vi "rd_data (WFM).vi"(4 "record index":u32, 6 "record info":T3, 7 "recordLenFromStart":u64, 8 "error in (no error)":errorcluster, 9 "length":u64, 10 "record start":u64, 11 "ExcelRefnum":T4) -> (0 "error out":errorcluster, 2 "data_AllTypeData":T1, 3 "real length":u64)   [LabVIEW 2020, in "NI_ExcelFile.lvlib"]
uses:
  <vilib>/express/express shared/NI_ExcelFile/NI_ExcelFile.lvlib
  <vilib>/express/express shared/NI_ExcelFile/Ctrls/ExcelRefnum.ctl
  <vilib>/express/express shared/NI_ExcelFile/Ctrls/MainData.ctl
  <vilib>/express/express shared/NI_ExcelFile/Ctrls/StreamMode.ctl
  <vilib>/express/express shared/NI_ExcelFile/Ctrls/TimeColumnMode.ctl
  <vilib>/express/express shared/NI_ExcelFile/Ctrls/FileAttribute.ctl
  <vilib>/express/express shared/NI_ExcelFile/Ctrls/Columns.ctl
  <vilib>/express/express shared/NI_ExcelFile/Ctrls/ColumnInfo.ctl
  <vilib>/express/express shared/NI_ExcelFile/Ctrls/DataType.ctl
  <vilib>/express/express shared/NI_ExcelFile/Ctrls/wd_recordInfo.ctl
  <vilib>/express/express shared/NI_ExcelFile/Ctrls/disk_TemplateFile.ctl
  <vilib>/express/express shared/NI_ExcelFile/Ctrls/meta_file.ctl
  <vilib>/express/express shared/NI_ExcelFile/Ctrls/meta_Block.ctl
  <vilib>/express/express shared/NI_ExcelFile/Ctrls/meta_BlockType.ctl
  <vilib>/express/express shared/NI_ExcelFile/Ctrls/data_AllTypeData.ctl
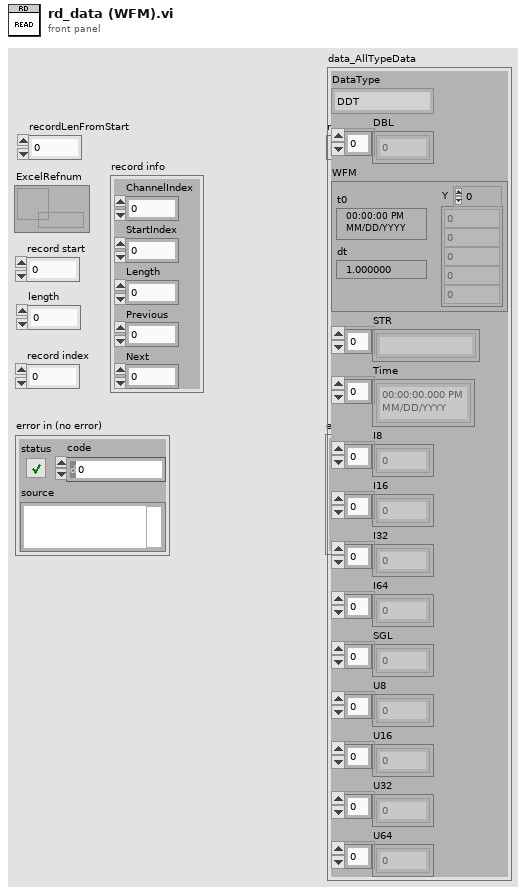
[diagram p1: front panel]
types:
  T1 = typedef "NI_ExcelFile.lvlib/data_AllTypeData.ctl" = cluster{"DataType":T2, "DBL":dbl[], "WFM":waveform(dbl), "STR":string[], "Time":timestamp[], "I8":i8[], "I16":i16[], "I32":i32[], "I64":i64[], "SGL":sgl[], "U8":u8[], "U16":u16[], "U32":u32[], "U64":u64[]}
  T2 = typedef "NI_ExcelFile.lvlib/DataType.ctl" = enum16{"DDT", "WFM", "Array of STR", "Array of DBL", "Array of I8", "Array of I16", "Array of I32", "Array of I64", "Array of SGL", "Array of U8", "Array of U16", "Array of U32", "Array of U64", "Array of Time"}
  T3 = typedef "NI_ExcelFile.lvlib/wd_recordInfo.ctl" = cluster{"ChannelIndex":u32, "StartIndex":u64, "Length":u64, "Previous":i32, "Next":i32}
  T4 = typedef "NI_ExcelFile.lvlib/ExcelRefnum.ctl" = refnum<data-value>
  T5 = typedef "NI_ExcelFile.lvlib/MainData.ctl" = cluster{"TargetFile":path, "StreamMode":T6, "Append?":bool, "ChunkSize":u64, "TimeColumnMode":T7, "TimestampFormat":string, "AbsoluteTime?":bool, "FileAttribute ":T8, "Column":T9, "FileRef":refnum<k1>, "MemoryRef":refnum<data-value>[], "RecordInfo":T3[], " ChannelPreviousInfo":u32[], "ChannelFirstRecord":u32[], "PredefinedFormattedValueLength":i64, "DiskTemplate":T11}
  T6 = typedef "NI_ExcelFile.lvlib/StreamMode.ctl" = enum16{"File", "Memory"}
  T7 = typedef "NI_ExcelFile.lvlib/TimeColumnMode.ctl" = enum16{"Empty", "OnePerCh", "One"}
  T8 = typedef "NI_ExcelFile.lvlib/FileAttribute.ctl" = cluster{"Creator":string, "Title":string, "SheetName":string}
  T9 = typedef "NI_ExcelFile.lvlib/Columns.ctl" = T10[]
  T10 = typedef "NI_ExcelFile.lvlib/ColumnInfo.ctl" = cluster{"Header":string, "Format":string, "DataType":T2, "Length":u64}
  T11 = typedef "NI_ExcelFile.lvlib/disk_TemplateFile.ctl" = cluster{"XMLRef":refnum<file>[], "ZipPath":path, "MetaFile":T12, "TempFolder":path}
  T12 = typedef "NI_ExcelFile.lvlib/meta_file.ctl" = cluster{"Ref":refnum<file>, "NextRow":i32, "NextPosition":i64, "Block":T13[]}
  T13 = typedef "NI_ExcelFile.lvlib/meta_Block.ctl" = cluster{"Version":u16, "Type":T14, "Length":i32, "Data":string}
  T14 = typedef "NI_ExcelFile.lvlib/meta_BlockType.ctl" = enum16{"NITag", "File", "Column"}
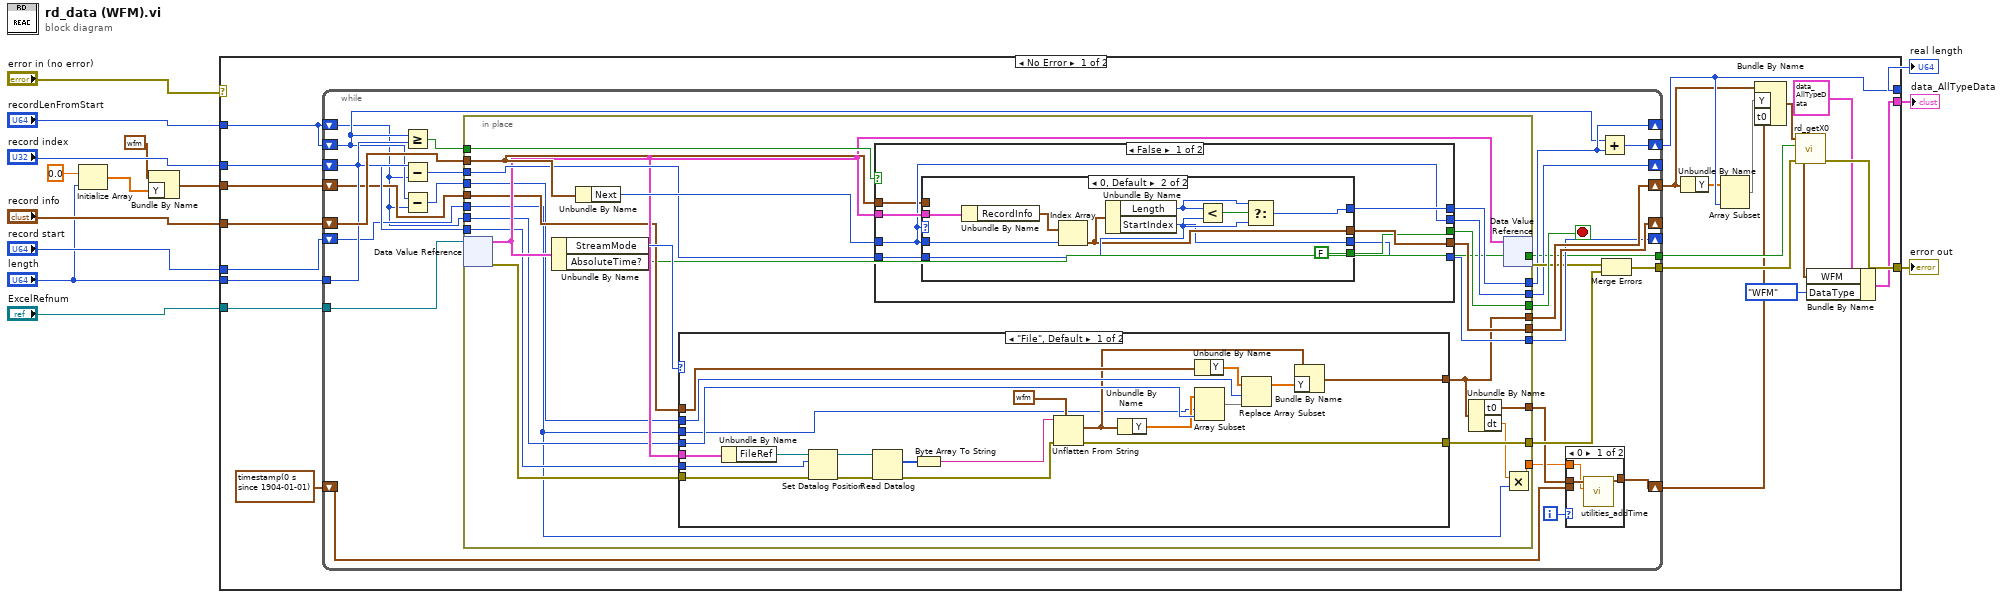
[diagram p0: block diagram]
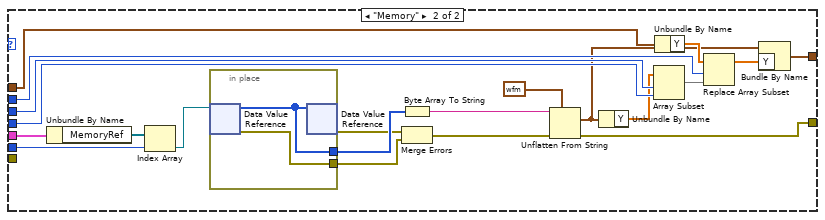
[diagram p3: hidden frame]
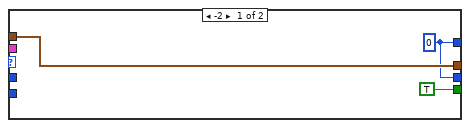
[diagram p4: hidden frame]
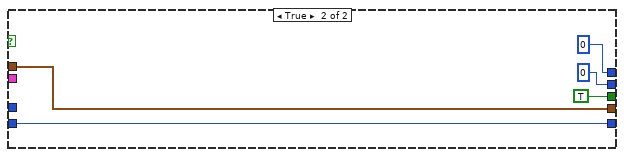
[diagram p5: hidden frame]
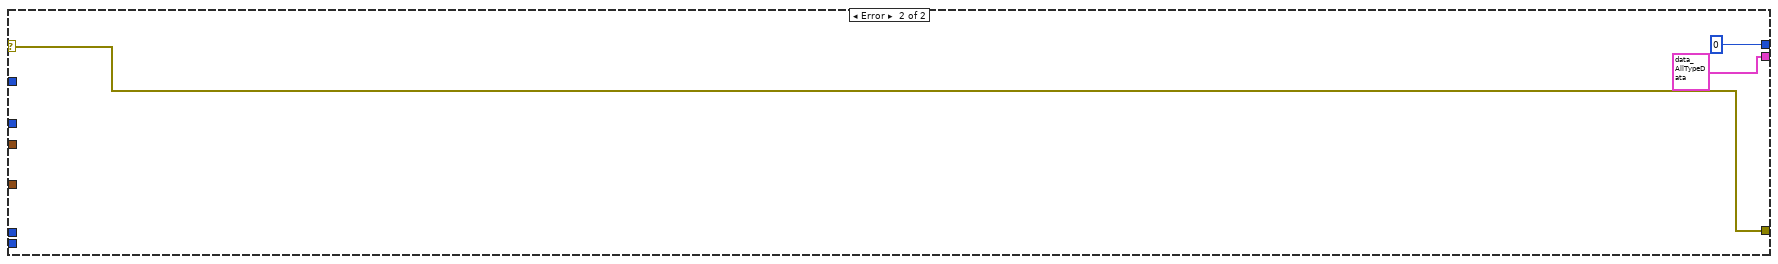
[diagram p6: hidden frame]
diagram:
  n1 = Initialize Array(0.0 ("element"), "length") -> (w4:dbl[])
  n2 = Bundle By Name(cluster=waveform(dbl) {"t0"=timestamp(0 s since 1904-01-01), "dt"=1.0, "Y"=[]} ("input waveform"), "Y"=w4) -> (w3:waveform(dbl))
  n3 = case shown="No Error" "error in (no error)" {
    selector: "error in (no error)" -> [_ w162]
    tunnel: [w18 T1 {"DataType"=enum."DDT", "DBL"=[], "WFM"={"t0"=timestamp(0 s since 1904-01-01), "dt"=1.0, "Y"=[]}, "STR"=[], "Time"=[], "I8"=[], "I16"=[], "I32"=[], "I64"=[], "SGL"=[], "U8"=[], "U16"=[], "U32"=[], "U64"=[]} ("fmt_AllTypeData")] -> w2
    tunnel: [w20 w162] -> w14
    tunnel: "record start" -> [w35 _]
    tunnel: "record index" -> [w31 _]
    tunnel: "ExcelRefnum" -> [w34 _]
    tunnel: "recordLenFromStart" -> [w30 _]
    tunnel: "length" -> [w33 _]
    tunnel: "record info" -> [w32 _]
    tunnel: [w29 u64 0 ("recordLenFromStart")] -> w9
    tunnel: w3 -> [w28 _]
    frame No Error {
      n4 = while {
        shift-right: [w45] -> _
        shift-left: w30 -> [w43]
        tunnel: w33 -> [w59]
        shift-right: [w60] -> _
        shift-left: w32 -> [w61]
        tunnel: w34 -> [w62]
        shift-right: [w57] -> w29
        shift-left: w30 -> [w44]
        shift-right: [w51] -> w26
        shift-left: w28 -> [w52]
        shift-right: [w46] -> _
        shift-left: w31 -> [w55]
        shift-right: [w50] -> _
        shift-left: w35 -> [w54]
        tunnel: [w47] -> w23
        tunnel: [w41] -> w22
        shift-right: [w39] -> w16
        shift-left: timestamp(0 s since 1904-01-01) ("Time out") -> [w37]
        i -> [w38]
        stop <- w53 stop-if-true
        n5 = Greater Or Equal?(x=w44, y=w59) -> (x >= y?=w56:bool)
        n6 = Subtract(x=w59, y=w43) -> (x-y=w58:u64)
        n7 = Subtract(x=w44, y=w43) -> (x-y=w42:u64)
        n8 = in-place {
          in-place-border: w61 -> [w88]
          in-place-border: w43 -> [w73]
          in-place-border: [w86] -> w60
          in-place-border: w58 -> [w85]
          in-place-border: [w84] -> w45
          in-place-border: w56 -> [w83]
          in-place-border: w55 -> [w80]
          in-place-border: w54 -> [w68]
          in-place-border: [w79] -> w46
          in-place-border: [w78] -> w53
          in-place-border: w52 -> [w77]
          in-place-border: [w71] -> w51
          in-place-border: [w76] -> w50
          in-place-border: [w75] -> w48
          in-place-border: w42 -> [w74]
          in-place-border: [w72] -> w41
          in-place-border: [w70] -> w40
          in-place-border: [w67] -> w36
          n9 = in-place-dvr #1(w62) -> (w81:T5, w89:errorcluster)
          n10 = Unbundle By Name(w81) -> ("StreamMode"=w82:T6, "AbsoluteTime?"=w72:bool)
          n11 = Unbundle By Name(w88) -> ("Next"=w87:i32)
          n12 = case shown="\"File\", Default" w82 {
            tunnel: w80 -> [w107 w128]
            tunnel: w89 -> [w106 _]
            tunnel: w68 -> [w90 w125]
            tunnel: w81 -> [w109 w131]
            tunnel: w77 -> [w93 w114]
            tunnel: [w92 w112] -> w71
            tunnel: [w101 w123] -> w75
            tunnel: w74 -> [w99 w119]
            tunnel: w73 -> [w98 w118]
            frame "File", Default {
              n13 = Unbundle By Name(w109) -> ("FileRef"=w108:refnum<k1>)
              n14 = Set Datalog Position(4:w106, 6:w107, 7:w108) -> (0:w105:errorcluster, 3:w110:refnum<k1>)  [unwired: 1 in]
              n15 = Read Datalog(4:w105, 7:w110) -> (0:w102:errorcluster, 2:w104:u8[])  [unwired: 1 in, 1 out]
              n16 = Byte Array To String(unsigned byte array=w104) -> (string=w103:string)
              n17 = Unflatten From String(type=waveform(dbl) {"t0"=timestamp(0 s since 1904-01-01), "dt"=1.0, "Y"=[]} ("input waveform"), binary string=w103, error in (no error)=w102) -> (value=w91:waveform(dbl), error out=w101:errorcluster)  [unwired: 2 in, 1 out]
              n18 = Unbundle By Name(w91) -> ("Y"=w96:dbl[])
              n19 = Unbundle By Name(w93) -> ("Y"=w95:dbl[])
              n20 = Array Subset(array=w96, index=w90, length=w98) -> (w100:dbl[])
              n21 = Replace Array Subset(array=w95, new element=w100, index=w99) -> (w94:dbl[])
              n22 = Bundle By Name(cluster=w91, "Y"=w94) -> (w92:waveform(dbl))
            }
            frame "Memory" {
              n23 = Unbundle By Name(w131) -> ("MemoryRef"=w129:refnum<data-value>[])
              n24 = Index Array(array=w129, index=w128) -> (element=w127:refnum<data-value>)
              n25 = in-place {
                in-place-border: [w133] -> w126
                in-place-border: [w132] -> w121
                n26 = in-place-dvr #2(w127) -> (w133:u8[], w132:errorcluster)
                n27 = in-place-dvr #2(w133) -> (w124:errorcluster)  [unwired: 1 out]
              }
              n28 = Byte Array To String(unsigned byte array=w126) -> (string=w130:string)
              n29 = Merge Errors(w124, w121) -> (w122:errorcluster)
              n30 = Unflatten From String(type=waveform(dbl) {"t0"=timestamp(0 s since 1904-01-01), "dt"=1.0, "Y"=[]} ("input waveform"), binary string=w130, error in (no error)=w122) -> (value=w111:waveform(dbl), error out=w123:errorcluster)  [unwired: 2 in, 1 out]
              n31 = Unbundle By Name(w111) -> ("Y"=w116:dbl[])
              n32 = Array Subset(array=w116, index=w125, length=w118) -> (w120:dbl[])
              n33 = Unbundle By Name(w114) -> ("Y"=w115:dbl[])
              n34 = Replace Array Subset(array=w115, new element=w120, index=w119) -> (w113:dbl[])
              n35 = Bundle By Name(cluster=w111, "Y"=w113) -> (w112:waveform(dbl))
            }
          }
          n36 = case shown="False" w83 {
            tunnel: w88 -> [w136 w157]
            tunnel: w87 -> [w137 _]
            tunnel: [w138 w157] -> w86
            tunnel: w85 -> [w139 w156]
            tunnel: [w141 u64 0 ("Length")] -> w84
            tunnel: w81 -> [w140 _]
            tunnel: [w137 u32 0 ("next")] -> w79
            tunnel: [w135 TRUE] -> w78
            tunnel: [w134 w156] -> w76
            frame False {
              n37 = case shown="0, Default" w137 {
                tunnel: [w142 w152] -> w141
                tunnel: w140 -> [_ w151]
                tunnel: w137 -> [_ w150]
                tunnel: w139 -> [_ w149]
                tunnel: [w144 w148] -> w138
                tunnel: w136 -> [w144 _]
                tunnel: [TRUE FALSE] -> w135
                tunnel: [w142 w146] -> w134
                frame -2 {
                  w142 = u64 0 ("Length")
                }
                frame 0, Default {
                  n38 = Unbundle By Name(w151) -> ("RecordInfo"=w154:T3[])
                  n39 = Index Array(array=w154, index=w150) -> (element=w148:T3)
                  n40 = Unbundle By Name(w148) -> ("Length"=w145:u64, "StartIndex"=w146:u64)
                  n41 = Less?(x=w145, y=w149) -> (x < y?=w153:bool)
                  n42 = Select(t=w145, s=w153, f=w149) -> (s? t:f=w152:u64)
                }
              }
            }
            frame True {
            }
          }
          n43 = Unbundle By Name(w71) -> ("t0"=w70:timestamp, "dt"=w69:dbl)
          n44 = in-place-dvr #1(w81) -> (w49:errorcluster)  [unwired: 1 out]
          n45 = Multiply(x=w69, y=w68) -> (x*y=w67:dbl)
        }
        n46 = case shown="0" w38 {
          tunnel: w40 -> [w65 _]
          tunnel: [w63 w66] -> w39
          tunnel: w37 -> [_ w66]
          tunnel: w36 -> [w64 _]
          frame 0 {
            n47 = call <vilib>:"utilities_addTime.vi"("number"=w64, "Time"=w65) -> ("Time out"=w63:timestamp)  [unwired: 9 in]
          }
          frame 1, Default {
          }
        }
        n48 = Add(x=w44, y=w45) -> (x+y=w57:u64)
        n49 = Merge Errors(w49, w48) -> (w47:errorcluster)
      }
      n50 = Unbundle By Name(w26) -> ("Y"=w27:dbl[])
      n51 = Array Subset(array=w27, length=w29) -> (w25:dbl[])  [unwired: 1 in]
      n52 = Bundle By Name(cluster=w26, "Y"=w25, "t0"=w16) -> (w24:waveform(dbl))
      n53 = call <vilib>:"rd_getX0.vi"("error in (no error)"=w23, "absolute time?"=w22, "WFM"=w24) -> ("error out"=w20:errorcluster, "WFM out"=w19:waveform(dbl))  [unwired: 7 in]
      n54 = Bundle By Name(cluster=T1 {"DataType"=enum."DDT", "DBL"=[], "WFM"={"t0"=timestamp(0 s since 1904-01-01), "dt"=1.0, "Y"=[]}, "STR"=[], "Time"=[], "I8"=[], "I16"=[], "I32"=[], "I64"=[], "SGL"=[], "U8"=[], "U16"=[], "U32"=[], "U64"=[]} ("fmt_AllTypeData"), "WFM"=w19, "DataType"=DataType."WFM") -> (w18:T1)
    }
    frame Error {
    }
  }
  "error out" <- w14
  "real length" <- w9
  "data_AllTypeData" <- w2
